vi "control.vi"(3 "from":T4, 4 "to":T4, 5 "operation_code":T4) -> (0 "operation":T2, 1 "regs_control":T3, 2 "alu_regs_control":T1)   [LabVIEW 2013]
panel:
  # "10000 for alu_first\n10001 for alu_second\n\n00100 for ax\n00101 for bx\n00110 for cx\n00111 for dx\n\n01000 for io"
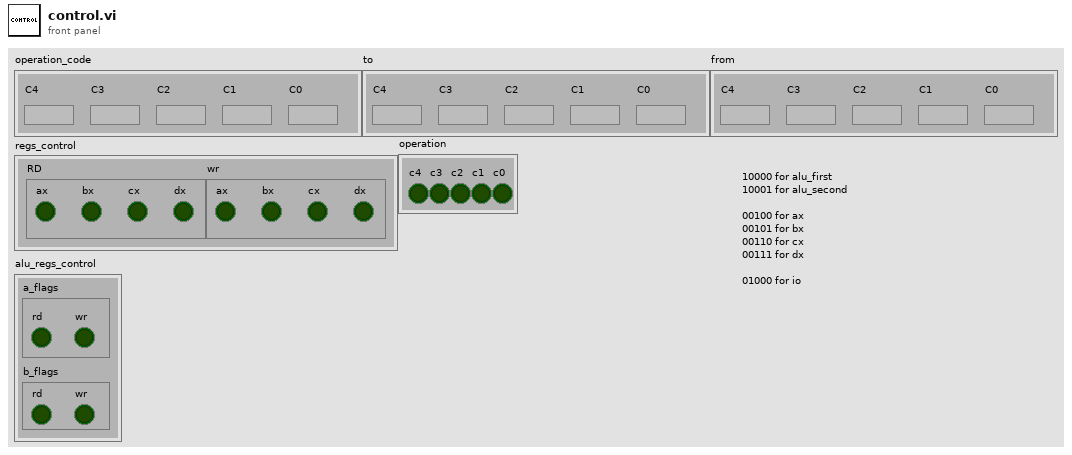
[diagram p1: front panel]
types:
  T1 = cluster{"a_flags":cluster{"rd":bool, "wr":bool}, "b_flags":cluster{"rd":bool, "wr":bool}}
  T2 = cluster{"c4":bool, "c3":bool, "c2":bool, "c1":bool, "c0":bool}
  T3 = cluster{"RD":cluster{"ax":bool, "bx":bool, "cx":bool, "dx":bool}, "wr":cluster{"ax":bool, "bx":bool, "cx":bool, "dx":bool}}
  T4 = cluster{"C4":bool, "C3":bool, "C2":bool, "C1":bool, "C0":bool}
  T5 = cluster{cluster{bool, bool}, cluster{bool, bool}}
  T6 = cluster{cluster{bool, bool, bool, bool}, cluster{bool, bool, bool, bool}}
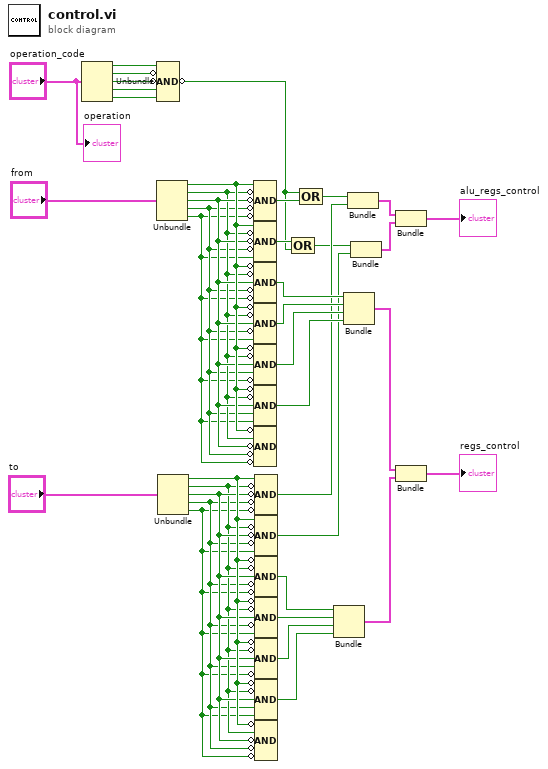
[diagram p0: block diagram]
diagram:
  n1 = Unbundle("operation_code") -> ("C4"=w39:bool, "C3"=w37:bool, "C2"=w38:bool, "C1"=w36:bool, "C0"=w35:bool)
  n2 = Compound Arithmetic op=AND(w39, invert w37, invert w38, w36, w35) -> (invert w1:bool)
  n3 = Unbundle("from") -> ("C4"=w31:bool, "C3"=w29:bool, "C2"=w30:bool, "C1"=w28:bool, "C0"=w27:bool)
  n4 = Unbundle("to") -> ("C4"=w26:bool, "C3"=w24:bool, "C2"=w25:bool, "C1"=w23:bool, "C0"=w22:bool)
  n5 = Compound Arithmetic op=AND(w31, invert w29, invert w30, invert w28, invert w27) -> (w2:bool)
  n6 = Compound Arithmetic op=AND(w31, invert w29, invert w30, invert w28, w27) -> (w5:bool)
  n7 = Compound Arithmetic op=AND(invert w31, invert w29, w30, invert w28, invert w27) -> (w18:bool)
  n8 = Compound Arithmetic op=AND(invert w31, invert w29, w30, invert w28, w27) -> (w17:bool)
  n9 = Compound Arithmetic op=AND(invert w31, invert w29, w30, w28, invert w27) -> (w16:bool)
  n10 = Compound Arithmetic op=AND(invert w31, invert w29, w30, w28, w27) -> (w15:bool)
  n11 = Compound Arithmetic op=AND(invert w31, w29, invert w30, invert w28, invert w27) -> ()  [unwired: 1 out]
  n12 = Compound Arithmetic op=AND(w26, invert w24, invert w25, invert w23, invert w22) -> (w10:bool)
  n13 = Compound Arithmetic op=AND(w26, invert w24, invert w25, invert w23, w22) -> (w9:bool)
  n14 = Compound Arithmetic op=AND(invert w26, invert w24, w25, invert w23, invert w22) -> (w14:bool)
  n15 = Compound Arithmetic op=AND(invert w26, invert w24, w25, invert w23, w22) -> (w13:bool)
  n16 = Compound Arithmetic op=AND(invert w26, invert w24, w25, w23, invert w22) -> (w12:bool)
  n17 = Compound Arithmetic op=AND(invert w26, invert w24, w25, w23, w22) -> (w11:bool)
  n18 = Compound Arithmetic op=AND(invert w26, w24, invert w25, invert w23, invert w22) -> ()  [unwired: 1 out]
  n19 = Compound Arithmetic op=OR(w5, w1) -> (w4:bool)
  n20 = Compound Arithmetic op=OR(w1, w2) -> (w3:bool)
  n21 = Bundle(w14, w13, w12, w11) -> (w19:cluster{bool, bool, bool, bool})  [unwired: 1 in]
  n22 = Bundle(w18, w17, w16, w15) -> (w20:cluster{bool, bool, bool, bool})  [unwired: 1 in]
  n23 = Bundle(w3, w10) -> (w8:cluster{bool, bool})  [unwired: 1 in]
  n24 = Bundle(w4, w9) -> (w7:cluster{bool, bool})  [unwired: 1 in]
  n25 = Bundle(w8, w7) -> (→"alu_regs_control":T5)  [unwired: 1 in]
  n26 = Bundle(w20, w19) -> (→"regs_control":T6)  [unwired: 1 in]
  "operation" <- "operation_code"
